vi "TriggerMode_SaveImagerA.vi"() -> ()   [LabVIEW 2022 SP3]
panel:
  in  "Stop Grabbing":bool
  out "# of Iteration":i32
  in  "ActiveFlyCapControl":refnum<k7>(container)
  # "This is an simlple ActiveX example using methods provided by ActiveFlyCapConctrol to grab images from an PGR camera,  \ndisplay it on the screen and retrieve the frame rate at the same time. Also, it can toggle between free running mode and software\ntrigger mode. It is meant to let new users become farmiliar with the ActiveX control provided by the Flycapture SDK, so more compilcated blocks can be build upon."
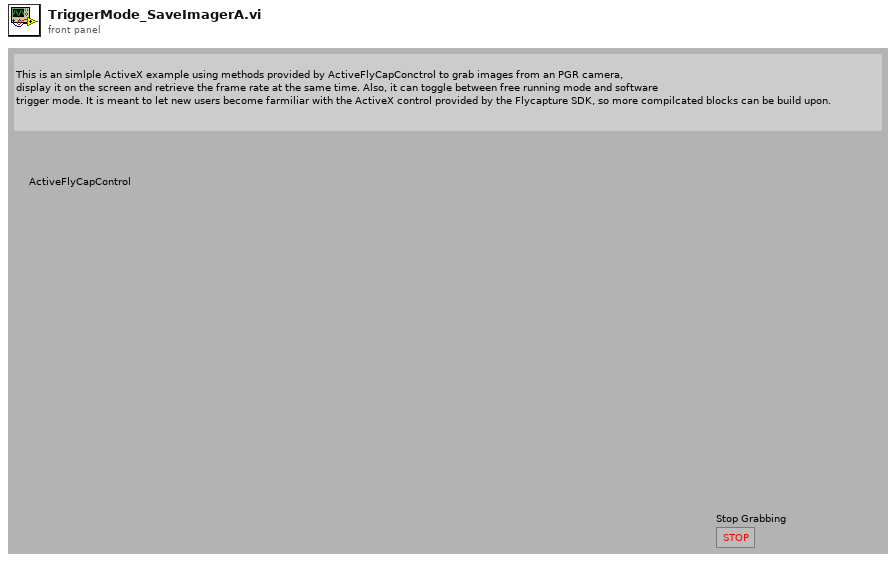
[diagram p1: front panel]
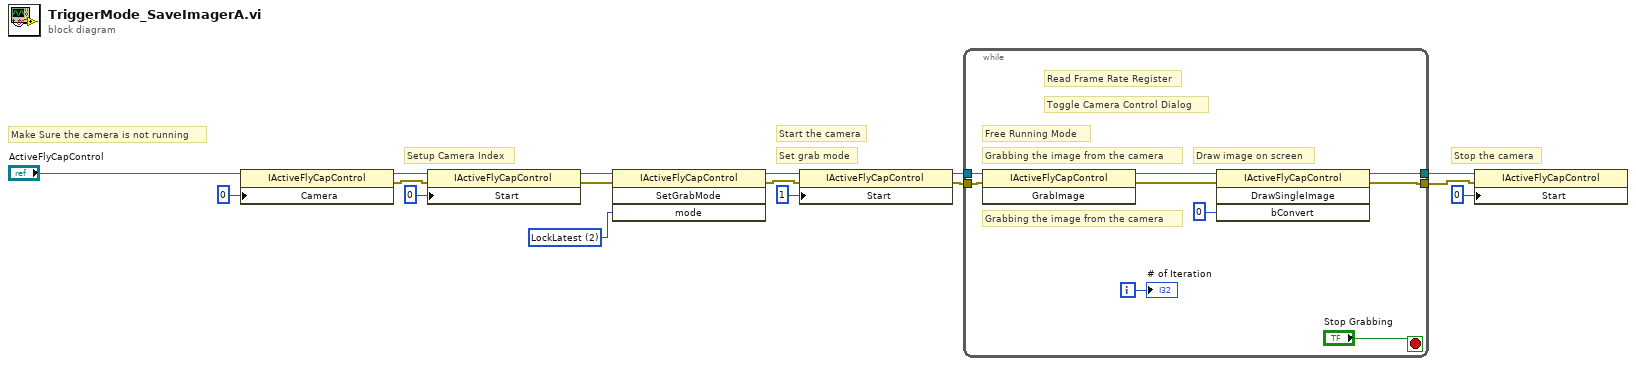
[diagram p0: block diagram]
diagram:
  w10 = 2 items=["FreeRunning", "LockNext", "LockLatest"] ("mode")
  # "Setup Camera Index"
  # "Set grab mode"
  # "Start the camera"
  # "Stop the camera"
  # "Make Sure the camera is not running"
  n1 = property class="IActiveFlyCapControl"(reference="ActiveFlyCapControl", "Camera"=0 ("Start")) -> (reference out=w7:refnum<k7>, error out=w4:errorcluster)  [unwired: 1 in]
  n2 = property class="IActiveFlyCapControl"(reference=w7, error in=w4, "Start"=0 ("Camera")) -> (reference out=w8:refnum<k7>, error out=w5:errorcluster)
  n3 = invoke class="IActiveFlyCapControl" method="SetGrabMode"(reference=w8, error in=w5, "mode"=w10) -> (reference out=w6:refnum<k7>, error out=w3:errorcluster)  [unwired: 1 in, 2 out]
  n4 = property class="IActiveFlyCapControl"(reference=w6, error in=w3, "Start"=1) -> (reference out=w11:refnum<k7>, error out=w2:errorcluster)
  n5 = while {
    tunnel: w11 -> [w22]
    tunnel: [w24] -> w12
    tunnel: w2 -> [w19]
    tunnel: [w17] -> w1
    i -> [w23]
    stop <- "Stop Grabbing" stop-if-true
    # "Draw image on screen"
    # "Grabbing the image from the camera"
    # "Grabbing the image from the camera"
    # "Free Running Mode"
    # "Read Frame Rate Register"
    # "Toggle Camera Control Dialog"
    n6 = invoke class="IActiveFlyCapControl" method="GrabImage"(reference=w22, error in=w19) -> (reference out=w21:refnum<k7>, error out=w18:errorcluster)  [unwired: 1 in, 1 out]
    n7 = invoke class="IActiveFlyCapControl" method="DrawSingleImage"(reference=w21, error in=w18, "bConvert"=0) -> (reference out=w24:refnum<k7>, error out=w17:errorcluster)  [unwired: 1 in, 2 out]
    "# of Iteration" <- w23
  }
  n8 = property class="IActiveFlyCapControl"(reference=w12, error in=w1, "Start"=0) -> ()  [unwired: 2 out]
